vi "Read Loop.vi"(8 "error in (no error)":errorcluster, 9 "ReadElements":u32, 10 "Queues":T1, 11 "AODAcq in":refnum<class "AODAcq.lvclass">) -> (0 "error out":errorcluster, 3 "AODAcq out":refnum<class "AODAcq.lvclass">)   [LabVIEW 2014, in "AODAcq.lvclass"]
uses:
  AODAcq.lvclass
panel:
  out "Progress":dbl(slide) scale=0.0..1.0
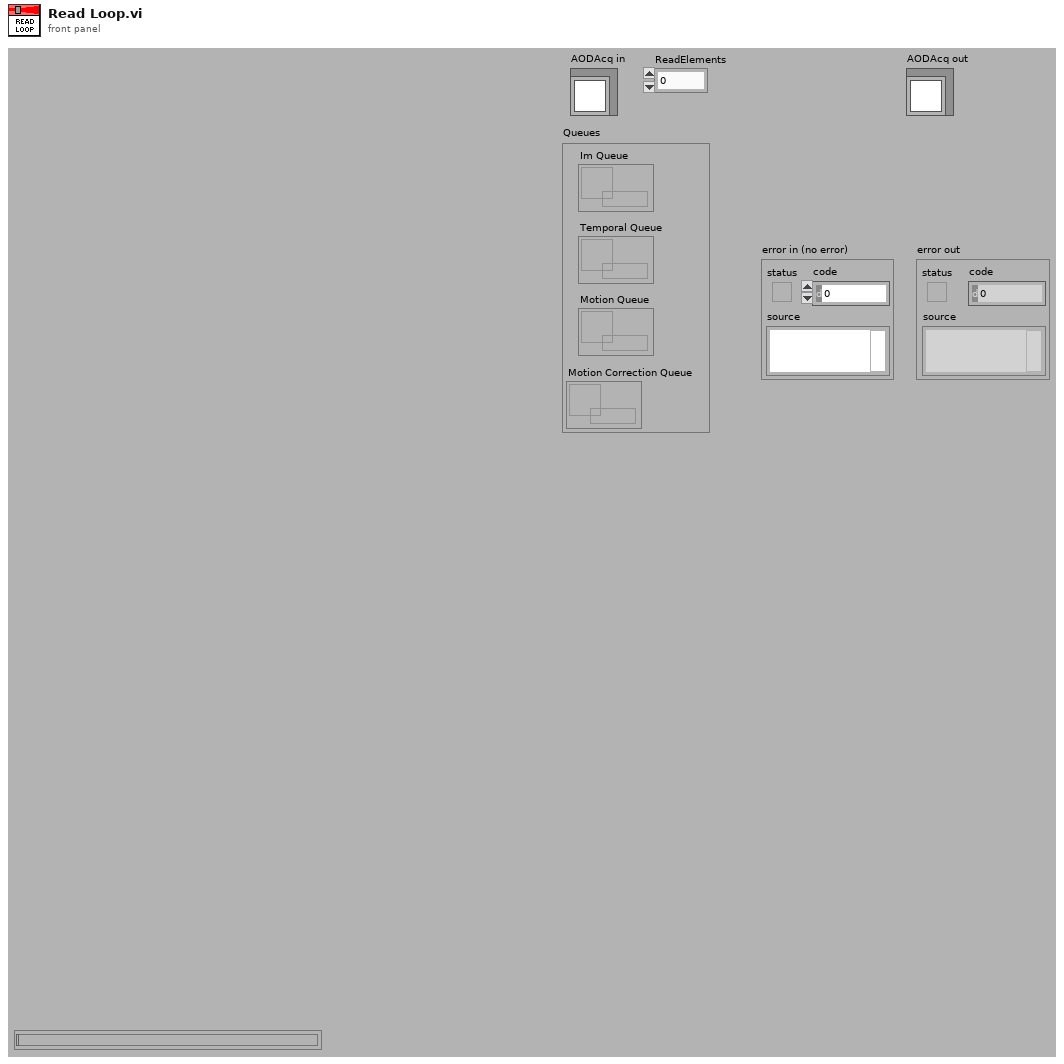
[diagram p1: front panel]
types:
  T1 = cluster{"Im Queue":refnum<queue>, "Temporal Queue":refnum<queue>, "Motion Queue":refnum<queue>, "Motion Correction Queue":refnum<queue>}
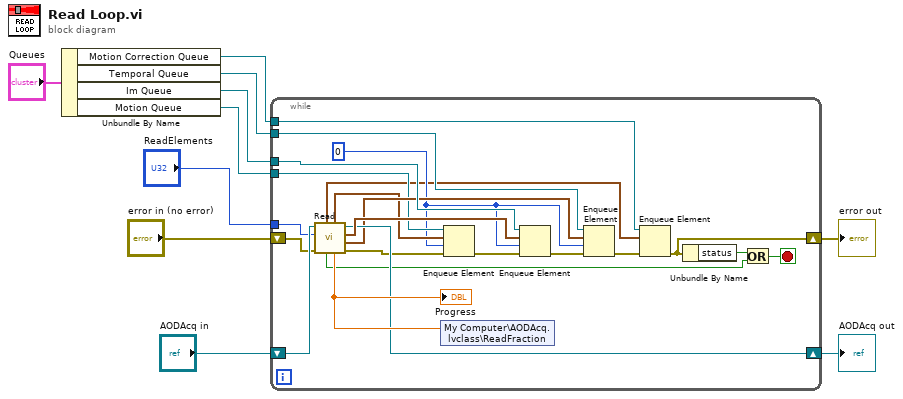
[diagram p0: block diagram]
diagram:
  n1 = Unbundle By Name("Queues") -> ("Motion Correction Queue"=w1:refnum<queue>, "Temporal Queue"=w3:refnum<queue>, "Im Queue"=w2:refnum<queue>, "Motion Queue"=w4:refnum<queue>)
  n2 = while {
    tunnel: w2 -> [w30]
    tunnel: "ReadElements" -> [w27]
    shift-right: [w24] -> w7
    shift-left: "AODAcq in" -> [w32]
    shift-right: [w14] -> w9
    shift-left: "error in (no error)" -> [w31]
    tunnel: w3 -> [w20]
    tunnel: w4 -> [w18]
    tunnel: w1 -> [w12]
    stop <- w25 stop-if-true
    w15 = 0 ("timeout in ms (-1)")
    n3 = call-dynamic "Read.vi"("error in (no error)"=w31, "ReadElements"=w27, "AODAcq in"=w32) -> ("error out"=w17:errorcluster, "TemporalData"=w21:waveform(dbl)[], "ImData"=w29:waveform(i32)[], "AODAcq out"=w24:refnum<class "AODAcq.lvclass">, "ReadFractionOut"=w28:dbl, "MotionData"=w19:waveform(i32)[], "Done"=w23:bool, "MotionCorrectionData"=w11:waveform(i32)[])  [unwired: 1 in]
    "Progress" <- w28
    n4 = shared-variable "My Computer\\AODAcq.lvclass\\ReadFraction"(w28) -> ()  [unwired: 1 in, 1 out]
    n5 = Enqueue Element(queue=w18, element=w19, timeout in ms (-1)=w15, error in (no error)=w17) -> (error out=w16:errorcluster)  [unwired: 2 out]
    n6 = Enqueue Element(queue=w30, element=w29, timeout in ms (-1)=w15, error in (no error)=w16) -> (error out=w22:errorcluster)  [unwired: 2 out]
    n7 = Enqueue Element(queue=w20, element=w21, timeout in ms (-1)=w15, error in (no error)=w22) -> (error out=w13:errorcluster)  [unwired: 2 out]
    n8 = Enqueue Element(queue=w12, element=w11, error in (no error)=w13) -> (error out=w14:errorcluster)  [unwired: 1 in, 2 out]
    n9 = Unbundle By Name(w14) -> ("status"=w26:bool)
    n10 = Or(x=w26, y=w23) -> (x .or. y?=w25:bool)
  }
  "error out" <- w9
  "AODAcq out" <- w7
